vi "Config.vi"(8 "error in (no error)":errorcluster, 10 "Setting":variant, 11 "Hioki BT4560B":refnum<class "Hioki BT4560B.lvclass">) -> (0 "error out":errorcluster, 3 "Hioki BT4560B out":refnum<class "Hioki BT4560B.lvclass">)   [LabVIEW 2025, in "ACIR.lvlib" / "Hioki BT4560B.lvclass"]
uses:
  Hioki BT4560B.lvclass
  C:/Users/Public/Documents/Sandia National Labs/TSS Plugin/CEF.lvlibp/Node/CEF_Node.lvclass
  C:/Working copy/tss/Plugin/Engines/ACIR/ACIR Instrument/ACIR Instrument.lvclass
  C:/Users/Public/Documents/Sandia National Labs/TSS Plugin/Abstract Engine.lvlibp/Plugin/Abstract/Abstract Instrument/Abstract Instrument.lvclass
  ACIR configuration/ACIR configuration.lvclass
  Hioki BT4560B.lvclass/Hioki BT4560B.ctl
  ACIR configuration/ACIR configuration.lvclass/ACIR configuration.ctl
  Users/Public/Documents/Sandia National Labs/TSS Plugin/Abstract Engine.lvlibp/Plugin/Abstract/Abstract Instrument/Channel.ctl
  ACIR Channel/ACIR Channel.lvclass
  Users/Public/Documents/Sandia National Labs/TSS Plugin/Abstract Engine.lvlibp/Plugin/Abstract/Channel configuration/Channel configuration.lvclass
  ACIR configuration/Read ACIR Setting.vi
  Users/Public/Documents/Sandia National Labs/TSS Plugin/CEF.lvlibp/Node/ReadChildren.vi
  Users/Public/Documents/Sandia National Labs/TSS Plugin/Abstract Engine.lvlibp/Plugin/Abstract/Channel configuration/Read Channel Setting.vi
  Users/Public/Documents/Sandia National Labs/TSS Plugin/CEF.lvlibp/Node/CEF_Node.lvclass
  Users/Public/Documents/Sandia National Labs/TSS Plugin/CEF.lvlibp/serializable configuration/CEF_serializable configuration.lvclass
  <instrlib>/HIOKI BT4560/HIOKI BT4560.lvlib
  Users/Public/Documents/Sandia National Labs/TSS Plugin/Abstract Engine.lvlibp/Plugin/Abstract/Abstract Instrument/Abstract Instrument.lvclass
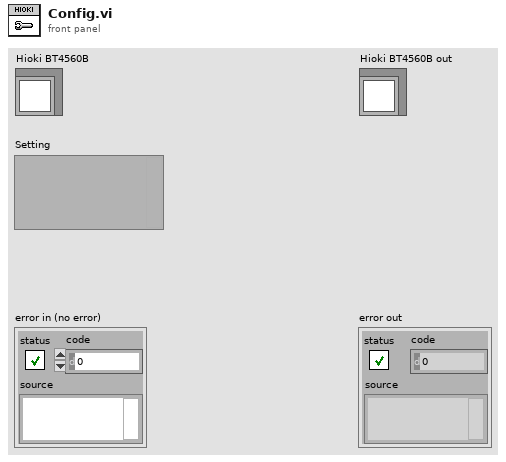
[diagram p1: front panel]
types:
  T1 = typedef "ACIR.lvlib/ACIR configuration.lvclass/ACIR Instrument Setting.ctl" = cluster{"Frequency":dbl, "Range":string, "Measurements":string}
  T2 = typedef "Abstract Engine.lvlibp/Abstract Instrument.lvclass/Channel.ctl" = cluster{"Alias":string, "DataType":enum16{"Anaolg Input", "Waveform"}, "Unit":enum16{"---", "V", "A", "Ohm", "Hz", "uF", "degC", "deg"}, "Upper limit":dbl, "Lower limit":dbl, "Measurement":variant}
  T3 = typedef "Abstract Engine.lvlibp/Channel configuration.lvclass/Default Channel.ctl" = cluster{"Address":string, "SW Alias":string, "Enabled":bool, "Type":string, "Description":string}
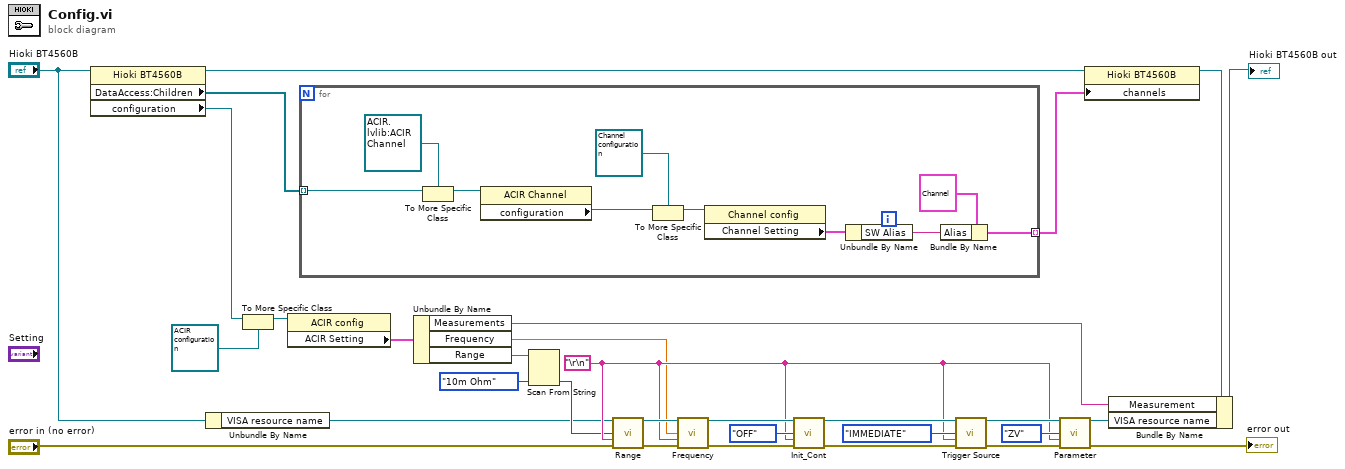
[diagram p0: block diagram]
diagram:
  w18 = "\r\n" ("End of Line Constant")
  n1 = property class="Hioki BT4560B"(reference="Hioki BT4560B") -> (reference out=w16:refnum<class "Hioki BT4560B.lvclass">, "DataAccess:Children"=w3:refnum<data-value>[], "configuration"=w4:refnum<class "CEF_serializable configuration.lvclass">)  [unwired: 1 in, 1 out]
  n2 = Unbundle By Name("Hioki BT4560B") -> ("VISA resource name"=w5:refnum<visa-resource-name>)
  n3 = To More Specific Class(target class=refnum<class "ACIR configuration.lvclass"> refnum ("Digitizer.lvlib:Digitizer configuration.lvclass"), reference=w4) -> (specific class reference=w8:refnum<class "ACIR configuration.lvclass">)  [unwired: 1 in, 1 out]
  n4 = property class="ACIR config"(reference=w8) -> ("ACIR Setting"=w7:T1)  [unwired: 1 in, 2 out]
  n5 = for {
    tunnel: w3 -> [w41] mode=indexing
    tunnel: [w38] -> w1 mode=indexing
    n6 = To More Specific Class(target class=refnum<data-value> refnum ("data value reference"), reference=w41) -> (specific class reference=w36:refnum<data-value>)  [unwired: 1 in, 1 out]
    n7 = property class="ACIR Channel"(reference=w36) -> ("configuration"=w35:refnum<class "CEF_serializable configuration.lvclass">)  [unwired: 1 in, 2 out]
    n8 = To More Specific Class(target class=refnum<class "Channel configuration.lvclass"> refnum ("Abstract Engine.lvlibp:Channel config"), reference=w35) -> (specific class reference=w33:refnum<class "Channel configuration.lvclass">)  [unwired: 1 in, 1 out]
    n9 = property class="Channel config"(reference=w33) -> ("Channel Setting"=w32:T3)  [unwired: 1 in, 2 out]
    n10 = Unbundle By Name(w32) -> ("SW Alias"=w39:string)
    n11 = Bundle By Name(cluster=T2 {"Alias"="ch0", "DataType"=enum."Anaolg Input", "Unit"=enum."V", "Upper limit"=10.0, "Lower limit"=-10.0, "Measurement"=variant(dbl 0.0)} ("Channel"), "Alias"=w39) -> (w38:T2)
  }
  n12 = Unbundle By Name(w7) -> ("Measurements"=w2:string, "Frequency"=w13:dbl, "Range"=w11:string)
  n13 = Scan From String(input string=w11, default 1=enum16{"3m Ohm", "10m Ohm", "100m Ohm"}."10m Ohm" ("Range set")) -> (output 1=w10:enum16{"3m Ohm", "10m Ohm", "100m Ohm"})  [unwired: 3 in, 3 out]
  n14 = call <instrlib>:"Range.vi"("VISA session"=w5, "Range set"=w10, "Terminator"=w18, "error in (no error)"="error in (no error)") -> ("dup VISA session"=w28:refnum<visa-resource-name>, "error out"=w27:errorcluster)  [unwired: 8 in, 2 out]
  n15 = call <instrlib>:"Frequency.vi"("VISA session"=w28, "Freq set"=w13, "Terminator"=w18, "error in (no error)"=w27) -> ("dup VISA session"=w21:refnum<visa-resource-name>, "error out"=w22:errorcluster)  [unwired: 8 in, 2 out]
  n16 = call <instrlib>:"Init_Cont.vi"("VISA session"=w21, "Cont Meas set"=enum16{"OFF", "ON"}."OFF", "Terminator"=w18, "error in (no error)"=w22) -> ("dup VISA session"=w20:refnum<visa-resource-name>, "error out"=w26:errorcluster)  [unwired: 8 in, 2 out]
  n17 = call <instrlib>:"Trigger Source.vi"("VISA session"=w20, "Trigger Source set"=enum16{"EXTERNAL", "IMMEDIATE"}."IMMEDIATE", "Terminator"=w18, "error in (no error)"=w26) -> ("dup VISA session"=w19:refnum<visa-resource-name>, "error out"=w25:errorcluster)  [unwired: 8 in, 2 out]
  n18 = call <instrlib>:"Parameter.vi"("VISA session"=w19, "Parameter set"=enum16{"RV", "ZV", "R", "Z", "V"}."ZV", "Terminator"=w18, "error in (no error)"=w25) -> ("dup VISA session"=w15:refnum<visa-resource-name>, "error out"=→"error out":errorcluster)  [unwired: 8 in, 2 out]
  n19 = property class="Hioki BT4560B"(reference=w16, "channels"=w1) -> (reference out=w9:refnum<class "Hioki BT4560B.lvclass">)  [unwired: 1 in, 1 out]
  n20 = Bundle By Name(cluster=w9, "Measurement"=w2, "VISA resource name"=w15) -> (→"Hioki BT4560B out":refnum<class "Hioki BT4560B.lvclass">)
